vi "ChemStation Control.vi"(10 "Command":string="LoadMethod \"C:\\Chem32\\1\\METHODS\\\"", 11 "ChemStation DDE name":string="hpcore7544") -> ()   [LabVIEW 2017]
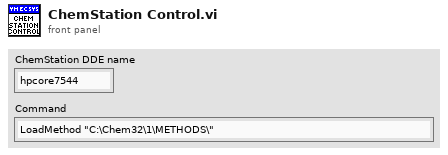
[diagram p1: front panel]
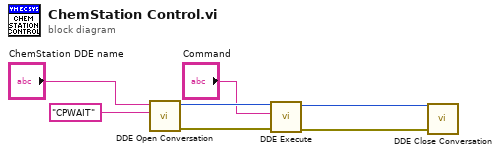
[diagram p0: block diagram]
diagram:
  n1 = call <vilib>:"DDE Open Conversation.vi"("topic"="CPWAIT", "service"="ChemStation DDE name") -> ("error out"=w4:errorcluster, "conversation refnum"=w5:u32)  [unwired: 6 in]
  n2 = call <vilib>:"DDE Execute.vi"("error in (no error)"=w4, "command"="Command", "conversation refnum in"=w5) -> ("error out"=w3:errorcluster, "conversation refnum out"=w2:u32)  [unwired: 5 in]
  n3 = call <vilib>:"DDE Close Conversation.vi"("error in (no error)"=w3, "conversation refnum"=w2) -> ()  [unwired: 7 in, 1 out]
